vi "Gen barcode.vi"(8 "error in (no error)":errorcluster, 10 "Full data":string[](array[string])) -> (0 "error out":errorcluster)   [LabVIEW 2020]
uses:
  <vilib>/Utility/sysdir.llb/System Directory Type.ctl
panel:
  out "new picture":picture
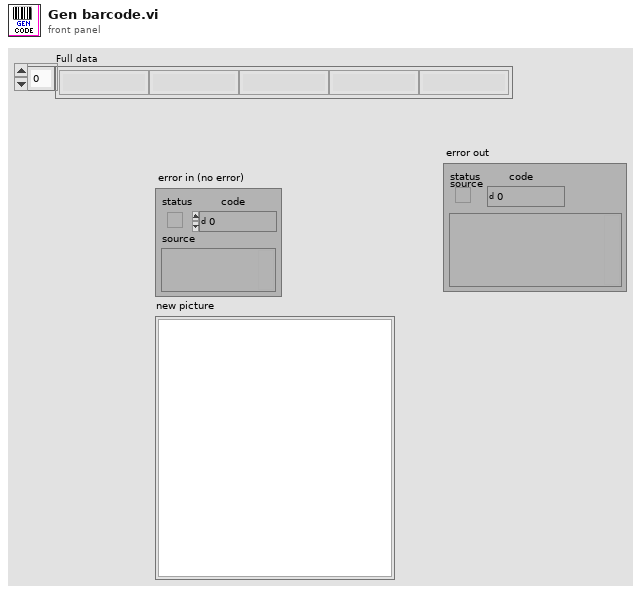
[diagram p1: front panel]
types:
  T1 = cluster{"horizontal":enum16{"left", "center", "right"}, "vertical":enum16{"top", "center", "bottom"}}
  T2 = enum16{"User-specified Font", "Application Font", "System Font", "Dialog Font"}
  T3 = cluster{"Font Name:":string, "Size":i16, "Strikeout?":bool, "Italic?":bool, "Underline?":bool, "Outline?":bool, "Shadow?":bool, "Bold?":bool}
  T4 = typedef "System Directory Type.ctl" = i32
  T5 = typedef "imagedata.ctl" = cluster{"image type":i32, "image depth":i32, "image":u8[], "mask":u8[], "colors":u32[], "Rectangle":cluster{"left":i16, "top":i16, "right":i16, "bottom":i16}}
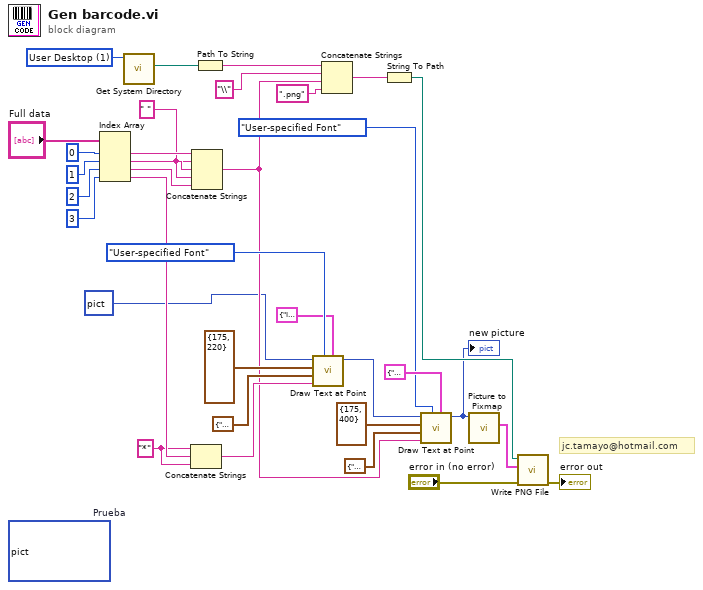
[diagram p0: block diagram]
diagram:
  w3 = " " ("string")
  (unwired) picture bytes[3000030]  # Prueba
  w6 = "*" ("string")
  w29 = T4 1 items=["User Home"=0, "User Desktop"=1, "User Documents"=2, "User Application Data"=3, "User Preferences"=4, "User Temporary"=5, "Public Documents"=6, "Public Application Data"=7, "Public Preferences"=8, "Public Cache"=13, "System Core Libraries"=9, "System Installed Libraries"=10, "Application Files"=11, "Boot Volume Root"=12] ("system directory type")
  # "jc.tamayo@hotmail.com"
  n1 = Index Array(array="Full data", index #1=0 ("index"), index #2=1 ("index"), index #3=2 ("index"), index #4=3 ("index")) -> (element #1=w5:string, element #2=w4:string, element #3=w2:string, element #4=w8:string)
  n2 = call <vilib>:"Get System Directory.vi"("system directory type"=w29) -> ("system directory"=w30:path)  [unwired: 10 in]
  n3 = Concatenate Strings(w6, w8, w6) -> (w15:string)
  n4 = Concatenate Strings(w5, w3, w4, w3, w2) -> (w9:string)
  n5 = Path To String(path=w30) -> (string=w28:string)
  n6 = call <vilib>:"Draw Text at Point.vi"("[user-specified font]"=T3 {"Font Name:"="IDAHC39M Code 39 Barcode", "Size"=170, "Strikeout?"=FALSE, "Italic?"=FALSE, "Underline?"=FALSE, "Outline?"=FALSE, "Shadow?"=FALSE, "Bold?"=FALSE}, "desired font(Application)"=T2."User-specified Font", "text"=w15, "alignment(left, top)"=T1 {"horizontal"=enum."center", "vertical"=enum."top"}, "origin"=cluster{"x":i16, "y":i16} {"x"=175, "y"=220}, "picture"=picture bytes[235596] ("new picture")) -> ("new picture"=w21:picture)  [unwired: 4 in, 1 out]
  n7 = Concatenate Strings(w28, "\\" ("string"), w9, ".png" ("string")) -> (w25:string)
  n8 = String To Path(string=w25) -> (path=w24:path)
  n9 = call <vilib>:"Draw Text at Point.vi"("[user-specified font]"=T3 {"Font Name:"="Adobe Gothic Std B", "Size"=48, "Strikeout?"=FALSE, "Italic?"=FALSE, "Underline?"=FALSE, "Outline?"=FALSE, "Shadow?"=FALSE, "Bold?"=FALSE}, "desired font(Application)"=T2."User-specified Font", "text"=w9, "alignment(left, top)"=T1 {"horizontal"=enum."center", "vertical"=enum."top"}, "origin"=cluster{"x":i16, "y":i16} {"x"=175, "y"=400}, "picture"=w21) -> ("new picture"=w16:picture)  [unwired: 4 in, 1 out]
  "new picture" <- w16
  n10 = call <vilib>:"Picture to Pixmap.vi"("picture"=w16) -> ("image data"=w31:T5)  [unwired: 9 in, 1 out]
  n11 = call <vilib>:"Write PNG File.vi"("error in (no error)"="error in (no error)", "image data"=w31, "path to PNG file"=w24) -> ("error out"=→"error out":errorcluster)  [unwired: 7 in, 1 out]
